vi "TestMoteComm.vi"() -> ()   [LabVIEW 2010]
uses:
  <vilib>/picture/picture.llb/Draw True-Color Pixmap.vi
panel:
  out "Counter Send/receive":dynamicdata(graph)
  out "Bytes written":i32
  out "Packet Sent":string
  in  "Enable Write":bool=TRUE
  out "bytes read":i32
  out "Packet Payload":string
  in  "Enable Read":bool=TRUE
  in  "Port Number":i32=9002
  out "KTH  Automatic Control \nTemplates. Test Bi-directional communication \nSerialForwarder-Mote":picture
  # "WRITE PACKET"
  # "READ PACKET"
  # "For TestSerialCommMsg:\nheaderSize = 9\npayload = 4"
  # "Communication control"
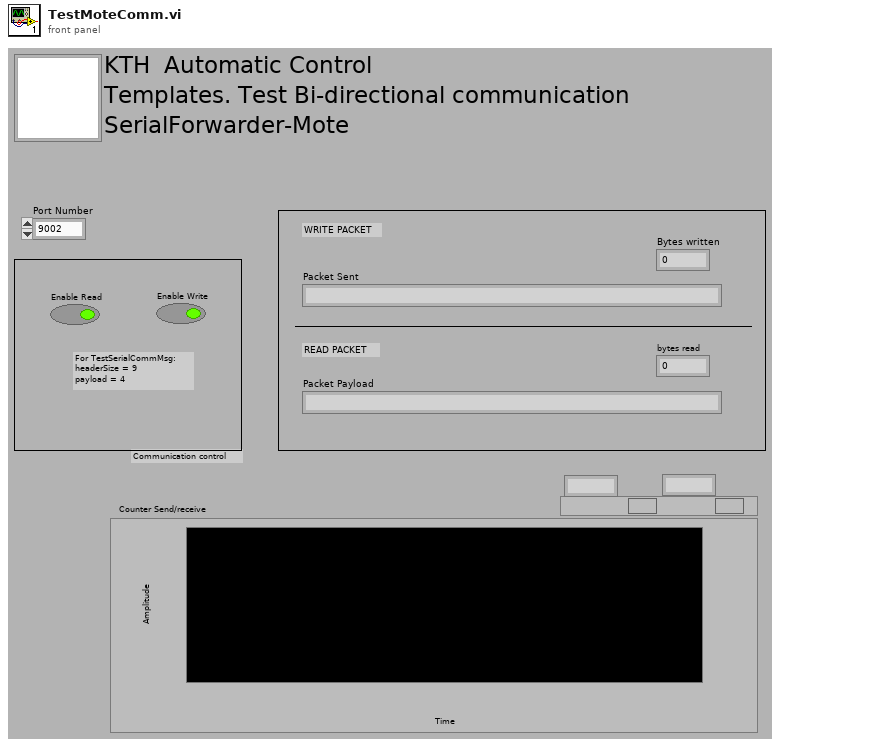
[diagram p1: front panel]
types:
  T1 = typedef "imagedata.ctl" = cluster{"image type":i32, "image depth":i32, "image":u8[], "mask":u8[], "colors":u32[], "Rectangle":cluster{"left":i16, "top":i16, "right":i16, "bottom":i16}}
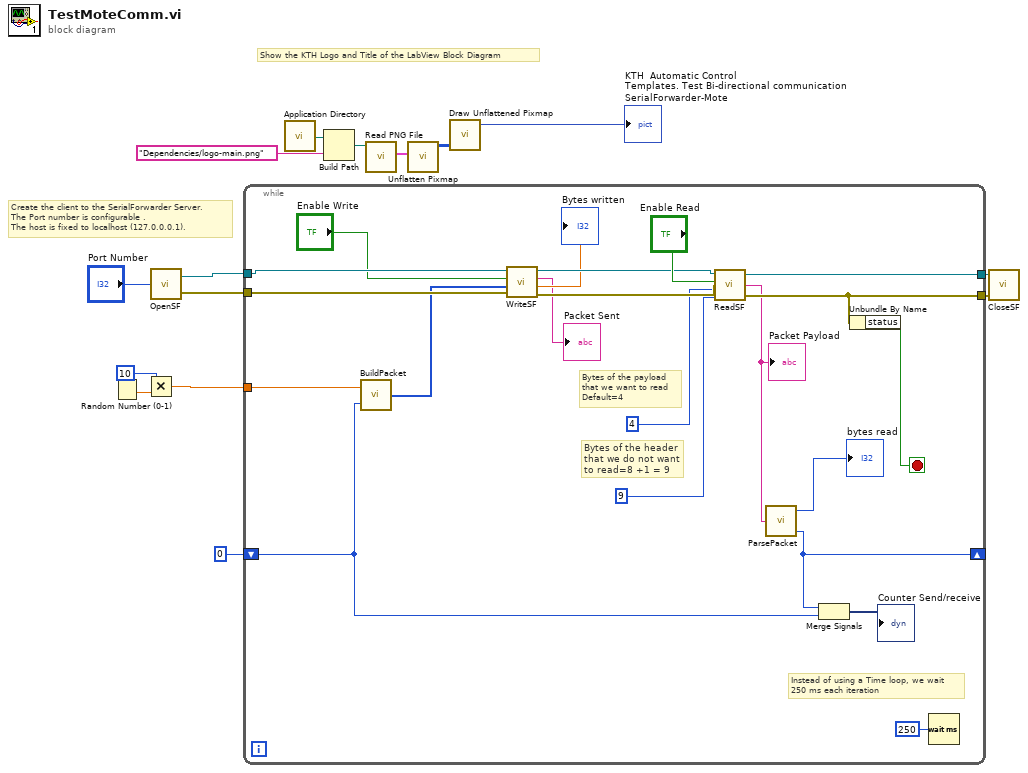
[diagram p0: block diagram]
diagram:
  # "Create the client to the SerialForwarder Server.\nThe Port number is configurable . \nThe host is fixed to localhost (127.0.0.0.1)."
  # "Show the KTH Logo and Title of the LabView Block Diagram"
  n1 = Random Number (0-1)() -> (number: 0 to 1=w3:dbl)
  n2 = Multiply(x=u16 10, y=w3) -> (x*y=w1:dbl)
  n3 = call "OpenSF.vi"("Port Number"="Port Number") -> ("error out"=w14:errorcluster, "connection ID"=w15:refnum<k5>)
  n4 = while {
    tunnel: w15 -> [w29]
    tunnel: w14 -> [w30]
    tunnel: [w36] -> w13
    tunnel: [w34] -> w12
    tunnel: w1 -> [w24]
    shift-right: [w18] -> _
    shift-left: u16 0 -> [w16]
    stop <- w35 stop-if-true
    # "Instead of using a Time loop, we wait \n250 ms each iteration"
    # "Bytes of the payload \nthat we want to read\nDefault=4"
    # "Bytes of the header\nthat we do not want \nto read=8 +1 = 9"
    n5 = call "BuildPacket.vi"("Counter"=w16, "Dummy"=w24) -> ("PacketArray"=w25:i32[])
    n6 = call "WriteSF.vi"("error in"=w30, "packet"=w25, "Enablle write"="Enable Write", "connection ID"=w29) -> ("error out"=w27:errorcluster, "Bytes written to SF"=→"Bytes written":dbl, "Packet String"=→"Packet Sent":string, "connection ID out"=w28:refnum<k5>)
    n7 = call "ReadSF.vi"("connection ID in"=w28, "enabled"="Enable Read", "bytes to read"=4, "header size"=9 ("bytes to read"), "error in"=w27) -> ("connection ID out"=w36:refnum<k5>, "string"=w32:string, "error out"=w34:errorcluster)
    "Packet Payload" <- w32
    n8 = call "ParsePacket.vi"("data out"=w32) -> ("Counter"=w18:i16, "Bytes read"=→"bytes read":i32)  [unwired: 1 out]
    n9 = Merge Signals(w18, w16) -> (→"Counter Send/receive":dynamicdata)
    n10 = Unbundle By Name(w34) -> ("status"=w35:bool)
    n11 = Wait (ms)(milliseconds to wait=u32 250) -> ()  [unwired: 1 out]
  }
  n12 = call <vilib>:"Application Directory.vi"() -> ("Application Directory"=w7:path)
  n13 = Build Path(base path=w7, name or relative path="Dependencies/logo-main.png") -> (appended path=w8:path)
  n14 = call <vilib>:"Read PNG File.vi"("path to PNG file"=w8) -> ("image data"=w11:T1)  [unwired: 8 in, 2 out]
  n15 = call <vilib>:"Unflatten Pixmap.vi"("image data"=w11) -> ("24-bit pixmap"=w10:u32[][])  [unwired: 4 in, 6 out]
  n16 = call-poly <vilib>:"Draw Unflattened Pixmap.vi"("data (RGB format)"=w10) -> ("new picture"=→"KTH  Automatic Control \nTemplates. Test Bi-directional communication \nSerialForwarder-Mote":picture)  [unwired: 8 in]
  n17 = call "CloseSF.vi"("error out"=w12, "connection ID"=w13) -> ()  [unwired: 1 in]
